vi "Set Position.vi"(8 "error in (no error)":errorcluster, 10 "Position":string, 11 "TrafficMap in":refnum<class "TrafficMap.lvclass">) -> (0 "error out":errorcluster, 3 "TrafficMap out":refnum<class "TrafficMap.lvclass">)   [LabVIEW 2017, in "TrafficMap.lvclass"]
uses:
  TrafficMap.lvclass
  TrafficMap.lvclass/TrafficMap.ctl
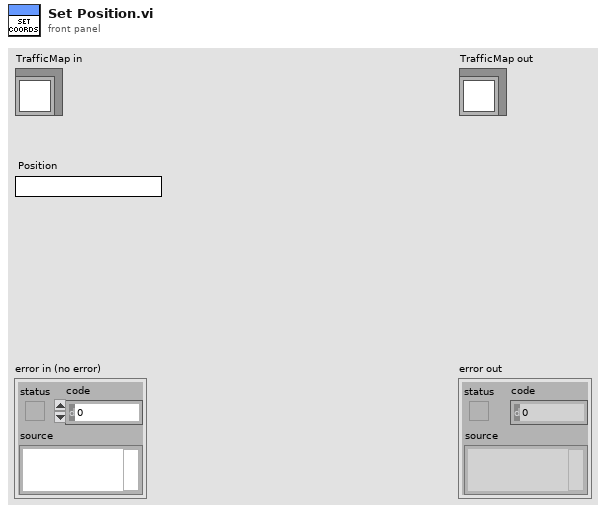
[diagram p1: front panel]
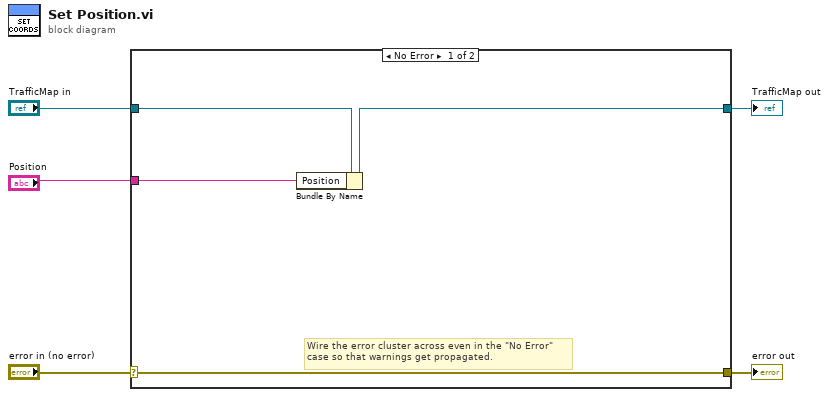
[diagram p0: block diagram]
diagram:
  n1 = case shown="No Error" "error in (no error)" {
    selector: "error in (no error)" -> [w9 w11]
    tunnel: [w9 w11] -> w4
    tunnel: [w6 w10] -> w2
    tunnel: "TrafficMap in" -> [w7 w10]
    tunnel: "Position" -> [w8 _]
    frame No Error {
      # "Wire the error cluster across even in the \"No Error\"\ncase so that warnings get propagated."
      n2 = Bundle By Name(cluster=w7, "Position"=w8) -> (w6:refnum<class "TrafficMap.lvclass">)
    }
    frame Error {
    }
  }
  "error out" <- w4
  "TrafficMap out" <- w2
